vi "Read Source.vi"(8 "Error In":errorcluster, 11 "Node In":refnum<class "Variable.lvclass">) -> (0 "Error Out":errorcluster, 2 "Source":string, 3 "Node Out":refnum<class "Variable.lvclass">)   [LabVIEW 2018, in "Toolkit.lvlib" / "Nodes.lvlib" / "Variable.lvclass"]
uses:
  Variable.lvclass
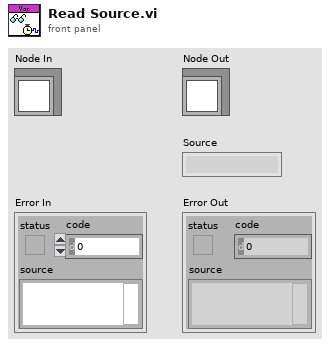
[diagram p1: front panel]
types:
  T1 = typedef "Toolkit.lvlib/Delimiters.ctl" = cluster{"Close":string, "Open":string}
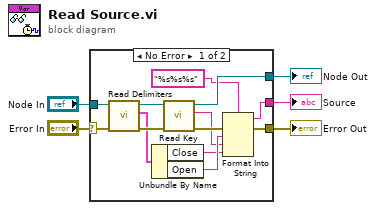
[diagram p0: block diagram]
diagram:
  n1 = case shown="No Error" "Error In" {
    selector: "Error In" -> [w6 w19]
    tunnel: "Node In" -> [w18 w20]
    tunnel: [w17 w20] -> w4
    tunnel: [w15 w19] -> w3
    tunnel: [w11 _] -> w2
    frame No Error {
      n2 = call-dynamic "Read Delimiters.vi"("Error In"=w6, "Node In"=w18) -> ("Error Out"=w13:errorcluster, "Delimiters"=w10:T1, "Node Out"=w14:refnum<class "Variable.lvclass">)  [unwired: 7 in]
      n3 = Unbundle By Name(w10) -> ("Close"=w7:string, "Open"=w9:string)
      n4 = call "Read Key.vi"("Error In"=w13, "Variable In"=w14) -> ("Error Out"=w16:errorcluster, "Key"=w8:string, "Variable Out"=w17:refnum<class "Variable.lvclass">)  [unwired: 7 in]
      n5 = Format Into String(format string="%s%s%s", error in=w16, w9, w8, w7) -> (resulting string=w11:string, error out=w15:errorcluster)  [unwired: 1 in]
    }
    frame Error {
    }
  }
  "Error Out" <- w3
  "Node Out" <- w4
  "Source" <- w2
